vi "DSP_init.vi"(1 "Initialize Instrument":u64=1024, 2 "Inst_param":T1={"Kind"=12, "Strings"=["Lock-in", "0:12", "V", "X;Y;Sensitivity", "V;V;a.u."], "uint64s"=[5, 19, 3, 0, 0, 0, 0, 1, 0, 27, 13, 2, 3], "Doubles"=[1.0, 0.10000000149011612, 37.70000076293945, 1.0, 0.0, 1000.0, 0.009999999776482582], "DAQmx take out list"=[]}) -> ()   [LabVIEW 2013]
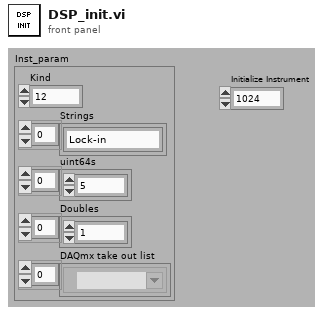
[diagram p1: front panel]
types:
  T1 = cluster{"Kind":u16, "Strings":string[], "uint64s":u64[], "Doubles":dbl[], "DAQmx take out list":refnum<k21>[]}
  T2 = enum16{"Signal_channel_coupling", "Signal_channel_input_mode", "SC_FET_BIPOLAR", "SC_LineFilter", "Auto_ac_gain", "AC_gain", "Sensitivity", "Auto_sensitivity", "Auto_phase", "Auto_sensitivity_phase", "Time_constant", "Reference_channel_source", "Oscillator_amplitude", "Oscilllator_frequency", "Parameter to be read"}[]
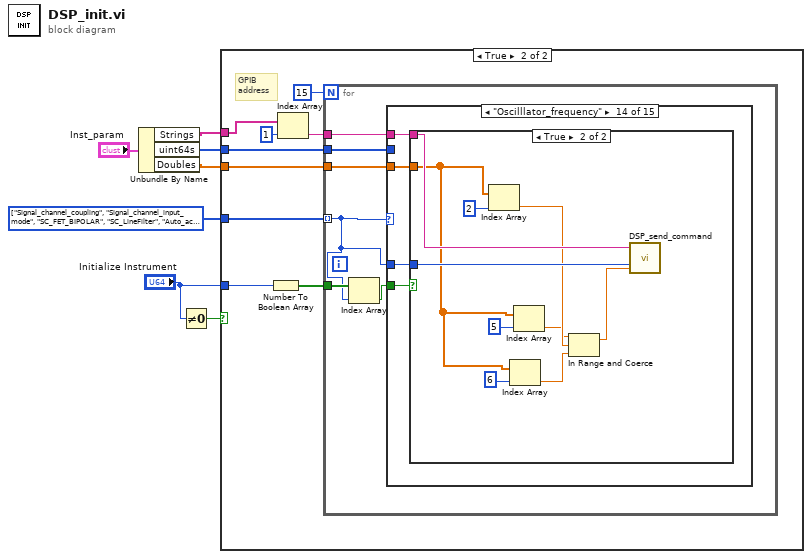
[diagram p0: block diagram]
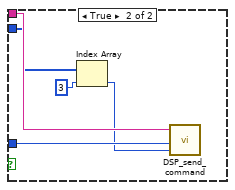
[diagram p4: hidden frame]
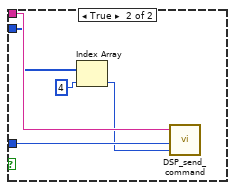
[diagram p6: hidden frame]
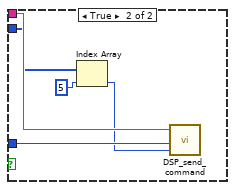
[diagram p8: hidden frame]
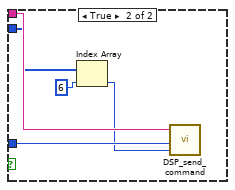
[diagram p10: hidden frame]
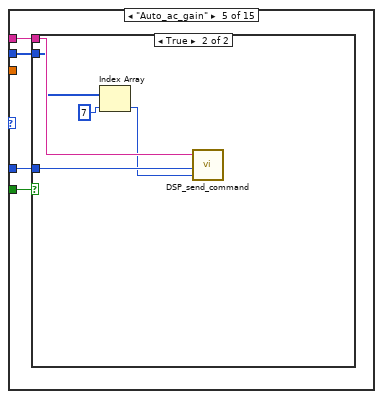
[diagram p11: hidden frame]
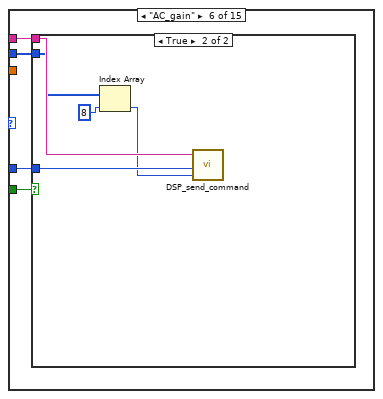
[diagram p13: hidden frame]
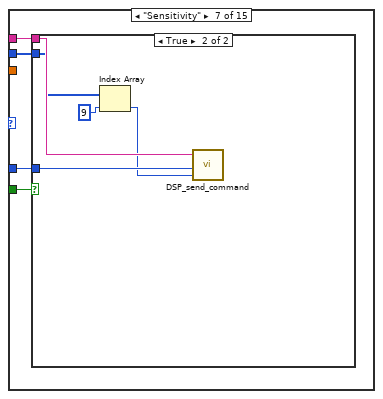
[diagram p15: hidden frame]
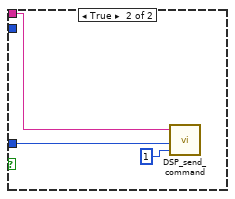
[diagram p18: hidden frame]
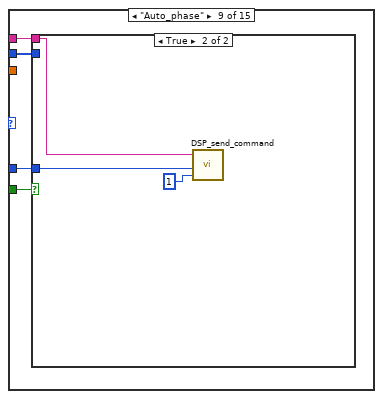
[diagram p19: hidden frame]
diagram:
  w1 = T2 [enum."Signal_channel_coupling", enum."Signal_channel_input_mode", enum."SC_FET_BIPOLAR", enum."SC_LineFilter", enum."Auto_ac_gain", enum."AC_gain", enum."Sensitivity", enum."Auto_sensitivity", enum."Auto_phase", enum."Auto_sensitivity_phase", enum."Time_constant", enum."Reference_channel_source", enum."Oscillator_amplitude", enum."Oscilllator_frequency", enum."Parameter to be read"] items=["Signal_channel_coupling", "Signal_channel_input_mode", "SC_FET_BIPOLAR", "SC_LineFilter", "Auto_ac_gain", "AC_gain", "Sensitivity", "Auto_sensitivity", "Auto_phase", "Auto_sensitivity_phase", "Time_constant", "Reference_channel_source", "Oscillator_amplitude", "Oscilllator_frequency", "Parameter to be read"]
  n1 = Unbundle By Name("Inst_param") -> ("Strings"=w5:string[], "uint64s"=w4:u64[], "Doubles"=w3:dbl[])
  n2 = Not Equal To 0?(x="Initialize Instrument") -> (x != 0?=w7:bool)
  n3 = case shown="True" w7 {
    tunnel: w5 -> [_ w11]
    tunnel: w4 -> [_ w10]
    tunnel: w3 -> [_ w9]
    tunnel: "Initialize Instrument" -> [_ w15]
    tunnel: w1 -> [_ w13]
    frame False {
    }
    frame True {
      # "GPIB\naddress"
      n4 = Number To Boolean Array(number=w15) -> (Boolean array=w14:bool[])
      n5 = Index Array(array=w11, index=1) -> (element=w8:string)
      n6 = for {
        N: 15 -> [_]
        tunnel: w14 -> [w19]
        tunnel: w13 -> [w17] mode=indexing
        tunnel: w10 -> [w22]
        tunnel: w9 -> [w21]
        tunnel: w8 -> [w20]
        n7 = Index Array(array=w19, index=w17) -> (element=w18:bool)
        n8 = case shown="\"Oscilllator_frequency\"" w17 {
          tunnel: w18 -> [w26 w35 w44 w53 w62 w71 w80 w89 w96 w103 w110 w119 w128 w142 w157]
          tunnel: w22 -> [w25 w34 w43 w52 w61 w70 w79 w88 w95 w102 w109 w118 _ _ w153]
          tunnel: w21 -> [_ _ _ _ _ _ _ _ _ _ _ _ w125 w139 w154]
          tunnel: w20 -> [w24 w33 w42 w51 w60 w69 w78 w87 w94 w101 w108 w117 w127 w141 w156]
          tunnel: w17 -> [w23 w32 w41 w50 w59 w68 w77 w86 w93 w100 w107 w116 w126 w140 w155]
          frame "Signal_channel_coupling", Default {
            n9 = case shown="False" w26 {
              tunnel: w25 -> [_ w29]
              tunnel: w24 -> [_ w31]
              tunnel: w23 -> [_ w30]
              frame False {
              }
              frame True {
                n10 = Index Array(array=w29, index=3) -> (element=w27:u64)
                n11 = call "DSP_send_command.vi"("Value"=w27, "CMD selection"=w30, "GPIB address"=w31) -> ()
              }
            }
          }
          frame "Signal_channel_input_mode" {
            n12 = case shown="False" w35 {
              tunnel: w34 -> [_ w38]
              tunnel: w33 -> [_ w40]
              tunnel: w32 -> [_ w39]
              frame False {
              }
              frame True {
                n13 = Index Array(array=w38, index=4) -> (element=w36:u64)
                n14 = call "DSP_send_command.vi"("Value"=w36, "CMD selection"=w39, "GPIB address"=w40) -> ()
              }
            }
          }
          frame "SC_FET_BIPOLAR" {
            n15 = case shown="False" w44 {
              tunnel: w43 -> [_ w47]
              tunnel: w42 -> [_ w49]
              tunnel: w41 -> [_ w48]
              frame False {
              }
              frame True {
                n16 = Index Array(array=w47, index=5) -> (element=w45:u64)
                n17 = call "DSP_send_command.vi"("Value"=w45, "CMD selection"=w48, "GPIB address"=w49) -> ()
              }
            }
          }
          frame "SC_LineFilter" {
            n18 = case shown="False" w53 {
              tunnel: w52 -> [_ w56]
              tunnel: w51 -> [_ w58]
              tunnel: w50 -> [_ w57]
              frame False {
              }
              frame True {
                n19 = Index Array(array=w56, index=6) -> (element=w54:u64)
                n20 = call "DSP_send_command.vi"("Value"=w54, "CMD selection"=w57, "GPIB address"=w58) -> ()
              }
            }
          }
          frame "Auto_ac_gain" {
            n21 = case shown="True" w62 {
              tunnel: w61 -> [_ w65]
              tunnel: w60 -> [_ w67]
              tunnel: w59 -> [_ w66]
              frame False {
              }
              frame True {
                n22 = Index Array(array=w65, index=7) -> (element=w63:u64)
                n23 = call "DSP_send_command.vi"("Value"=w63, "CMD selection"=w66, "GPIB address"=w67) -> ()
              }
            }
          }
          frame "AC_gain" {
            n24 = case shown="True" w71 {
              tunnel: w70 -> [_ w74]
              tunnel: w69 -> [_ w76]
              tunnel: w68 -> [_ w75]
              frame False {
              }
              frame True {
                n25 = Index Array(array=w74, index=8) -> (element=w72:u64)
                n26 = call "DSP_send_command.vi"("Value"=w72, "CMD selection"=w75, "GPIB address"=w76) -> ()
              }
            }
          }
          frame "Sensitivity" {
            n27 = case shown="True" w80 {
              tunnel: w79 -> [_ w83]
              tunnel: w78 -> [_ w85]
              tunnel: w77 -> [_ w84]
              frame False {
              }
              frame True {
                n28 = Index Array(array=w83, index=9) -> (element=w81:u64)
                n29 = call "DSP_send_command.vi"("Value"=w81, "CMD selection"=w84, "GPIB address"=w85) -> ()
              }
            }
          }
          frame "Auto_sensitivity" {
            n30 = case shown="False" w89 {
              tunnel: w88 -> [_ _]
              tunnel: w87 -> [_ w92]
              tunnel: w86 -> [_ w91]
              frame False {
              }
              frame True {
                n31 = call "DSP_send_command.vi"("Value"=1, "CMD selection"=w91, "GPIB address"=w92) -> ()
              }
            }
          }
          frame "Auto_phase" {
            n32 = case shown="True" w96 {
              tunnel: w95 -> [_ _]
              tunnel: w94 -> [_ w99]
              tunnel: w93 -> [_ w98]
              frame False {
              }
              frame True {
                n33 = call "DSP_send_command.vi"("Value"=1, "CMD selection"=w98, "GPIB address"=w99) -> ()
              }
            }
          }
          frame "Auto_sensitivity_phase" {
            n34 = case shown="False" w103 {
              tunnel: w102 -> [_ _]
              tunnel: w101 -> [_ w106]
              tunnel: w100 -> [_ w105]
              frame False {
              }
              frame True {
                n35 = call "DSP_send_command.vi"("Value"=1, "CMD selection"=w105, "GPIB address"=w106) -> ()
              }
            }
          }
          frame "Time_constant" {
            n36 = case shown="True" w110 {
              tunnel: w109 -> [_ w112]
              tunnel: w108 -> [_ w115]
              tunnel: w107 -> [_ w114]
              frame False {
              }
              frame True {
                n37 = Index Array(array=w112, index=10) -> (element=w111:u64)
                n38 = call "DSP_send_command.vi"("Value"=w111, "CMD selection"=w114, "GPIB address"=w115) -> ()
              }
            }
          }
          frame "Reference_channel_source" {
            n39 = case shown="True" w119 {
              tunnel: w118 -> [_ w121]
              tunnel: w117 -> [_ w124]
              tunnel: w116 -> [_ w123]
              frame False {
              }
              frame True {
                n40 = Index Array(array=w121, index=11) -> (element=w120:u64)
                n41 = call "DSP_send_command.vi"("Value"=w120, "CMD selection"=w123, "GPIB address"=w124) -> ()
              }
            }
          }
          frame "Oscillator_amplitude" {
            n42 = case shown="True" w128 {
              tunnel: w127 -> [_ w138]
              tunnel: w126 -> [_ w137]
              tunnel: w125 -> [_ w133]
              frame False {
              }
              frame True {
                n43 = Index Array(array=w133, index=1) -> (element=w130:dbl)
                n44 = Index Array(array=w133, index=4) -> (element=w131:dbl)
                n45 = Index Array(array=w133, index=3) -> (element=w132:dbl)
                n46 = In Range and Coerce(upper limit=w132, x=w130, lower limit=w131) -> (coerced(x)=w129:dbl)  [unwired: 1 out]
                n47 = call "DSP_send_command.vi"("Value"=w129, "CMD selection"=w137, "GPIB address"=w138) -> ()
              }
            }
          }
          frame "Oscilllator_frequency" {
            n48 = case shown="True" w142 {
              tunnel: w141 -> [_ w152]
              tunnel: w140 -> [_ w151]
              tunnel: w139 -> [_ w144]
              frame False {
              }
              frame True {
                n49 = Index Array(array=w144, index=2) -> (element=w147:dbl)
                n50 = Index Array(array=w144, index=6) -> (element=w145:dbl)
                n51 = Index Array(array=w144, index=5) -> (element=w146:dbl)
                n52 = In Range and Coerce(upper limit=w146, x=w147, lower limit=w145) -> (coerced(x)=w143:dbl)  [unwired: 1 out]
                n53 = call "DSP_send_command.vi"("Value"=w143, "CMD selection"=w151, "GPIB address"=w152) -> ()
              }
            }
          }
          frame "Parameter to be read" {
            n54 = case shown="True" w157 {
              tunnel: w156 -> [_ w159]
              tunnel: w155 -> [_ _]
              tunnel: w154 -> [_ _]
              tunnel: w153 -> [_ w158]
              frame False {
              }
              frame True {
                n55 = Index Array(array=w158, index=1) -> (element=w161:u64)
                n56 = Number To Decimal String(number=w161) -> (decimal integer string=w163:string)  [unwired: 1 in]
                n57 = Concatenate Strings("CBD ", w163) -> (w160:string)
                n58 = GPIB Write(0:w159, 1:w160) -> ()  [unwired: 3 in, 2 out]
              }
            }
          }
        }
      }
    }
  }
